vi "Current_Training_UI_3.10.22.vi"() -> ()   [LabVIEW 2019]
panel:
  out "Console out 2":string
  out "Console out":string
  out "intro":picture
  out "view":picture
  out "training 2":picture
  out "sent string":string
  out "training":u16[](array[numeric])
  out "Motor Value":i32
  in  "Quit":bool
  out "Training String":string
  out "Tab Control":enum32{"Welcome", "View", "Train"}(tab)
  in  "Ready":bool
  out "Motor Position View":u8(knob) scale=0.0..4.0
  in  "TRAIN":bool
  out "Sensor Intensity % View":dbl(slide) scale=0.0..100.0
  out "?":u32(colorbox)
  in  "Done":bool
  in  "Motor Position":u8(knob) scale=0.0..4.0
  out "Light Intensity %":dbl(slide) scale=0.0..100.0
  in  "Training Data":bool
  in  "Upload":bool
  out "Light Intensity 2":u32(colorbox)
  out "table":picture
  in  "Done 2":bool
  out "concatenated string":string
  out "read buffer":string
  out "Motor":string
  out "Sensor":string
  out "Type":string
  out "Name":string
  out "read terminal buffer - view":string
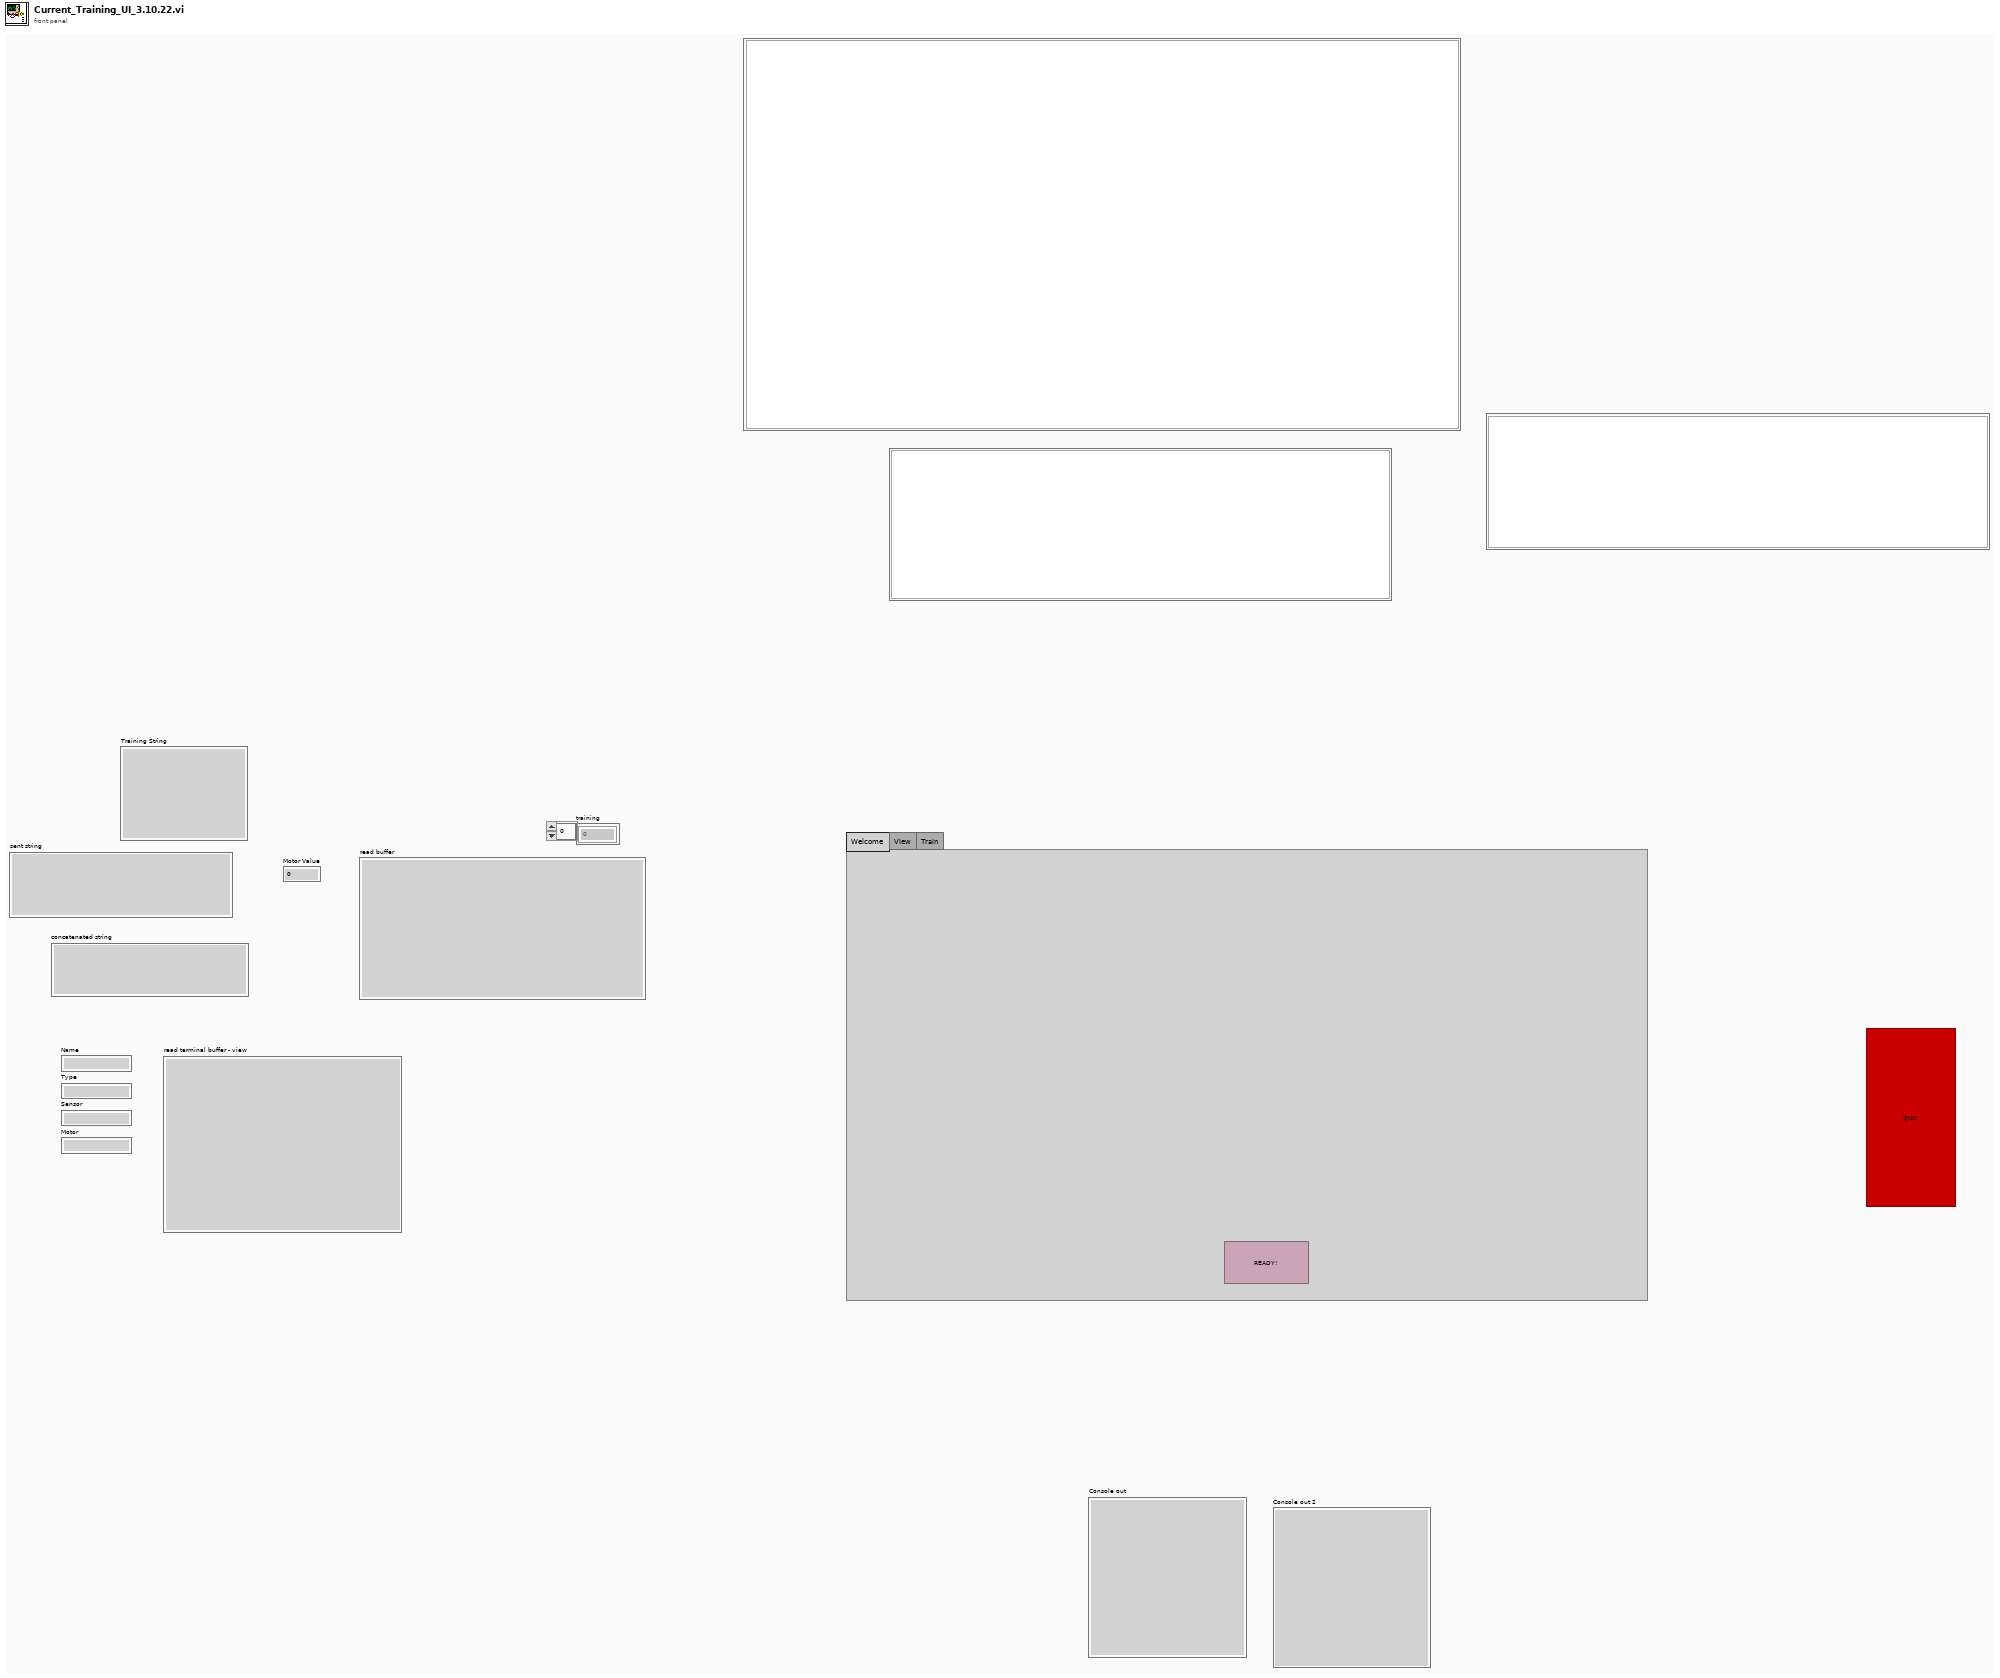
[diagram p1: front panel]
types:
  T1 = typedef "PythonCtrl.ctl" = cluster{"session":refnum<k35>, "PyPath":path, "Processor":enum16{"SPIKE", "Pi", "Pi_ssh"}}
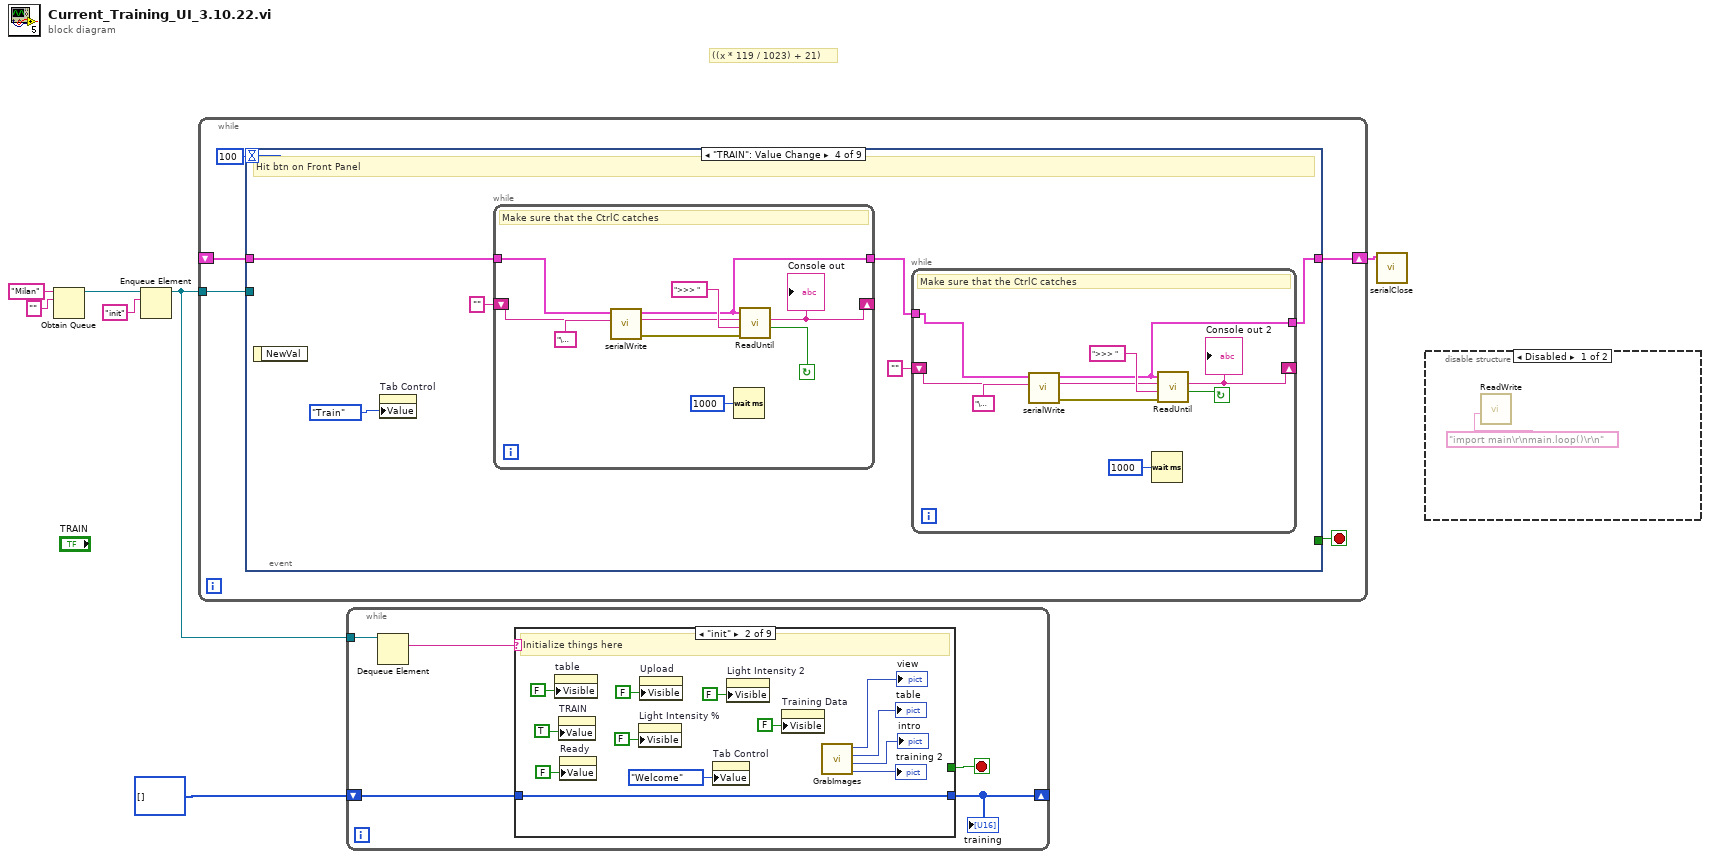
[diagram p0: block diagram]
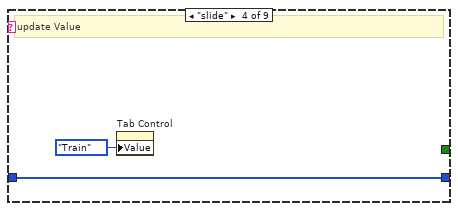
[diagram p5: hidden frame]
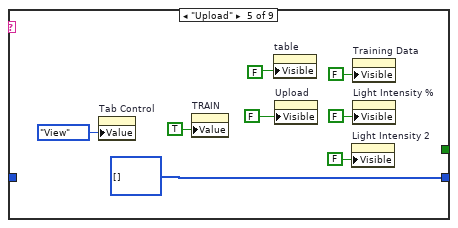
[diagram p6: hidden frame]
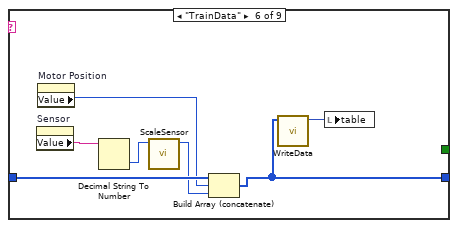
[diagram p7: hidden frame]
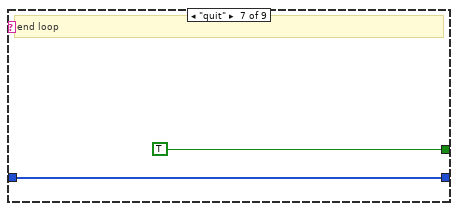
[diagram p8: hidden frame]
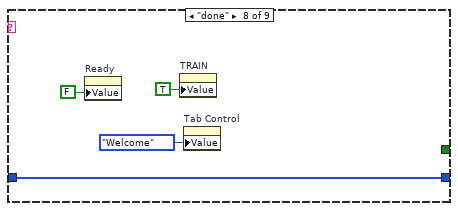
[diagram p9: hidden frame]
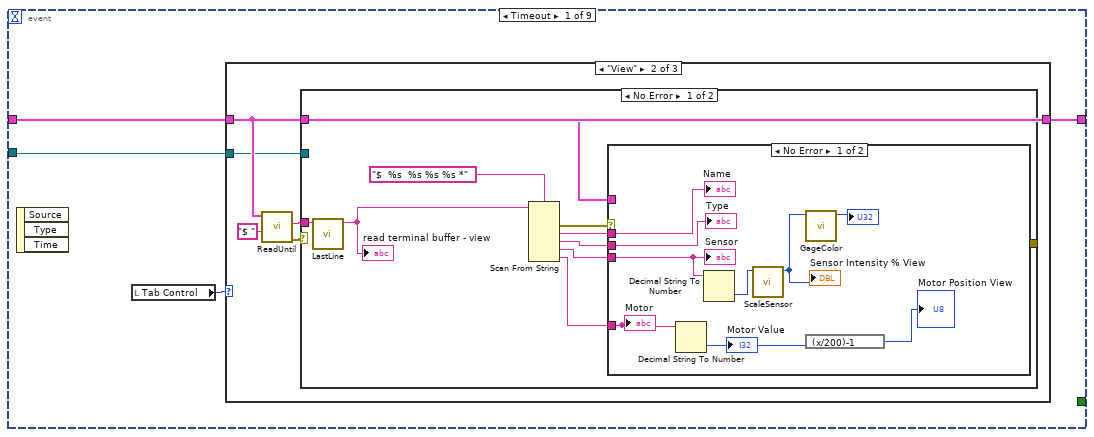
[diagram p11: hidden frame]
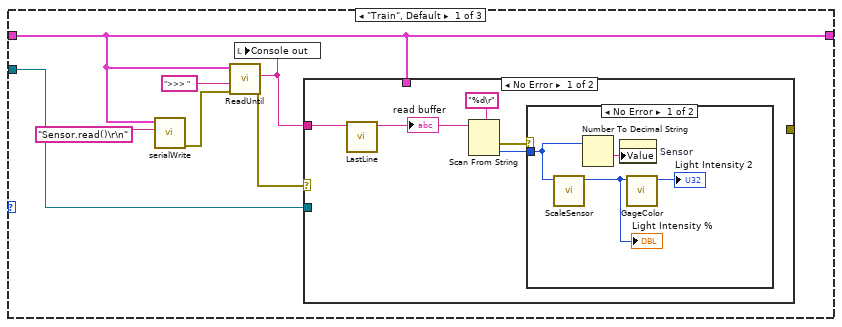
[diagram p12: hidden frame]
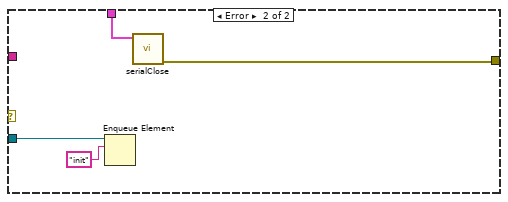
[diagram p14: hidden frame]
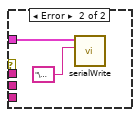
[diagram p15: hidden frame]
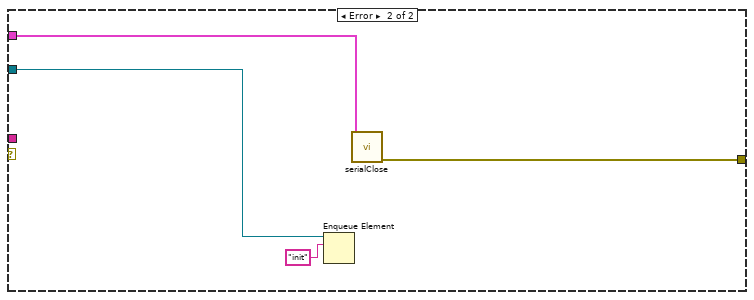
[diagram p16: hidden frame]
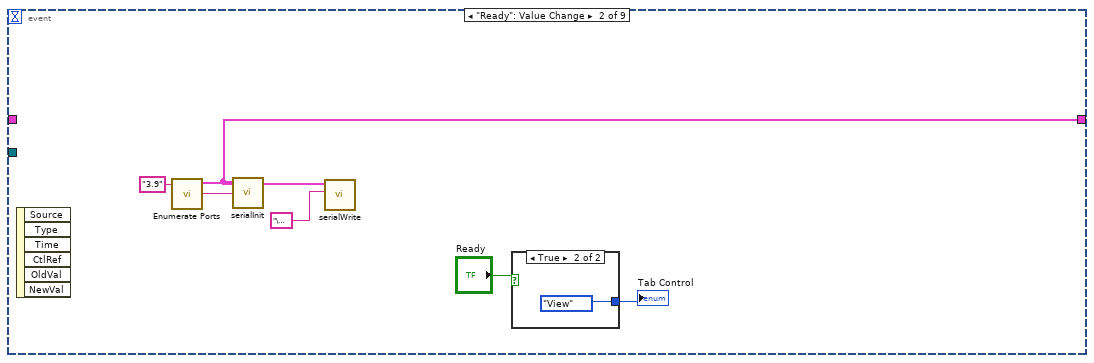
[diagram p18: hidden frame]
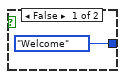
[diagram p19: hidden frame]
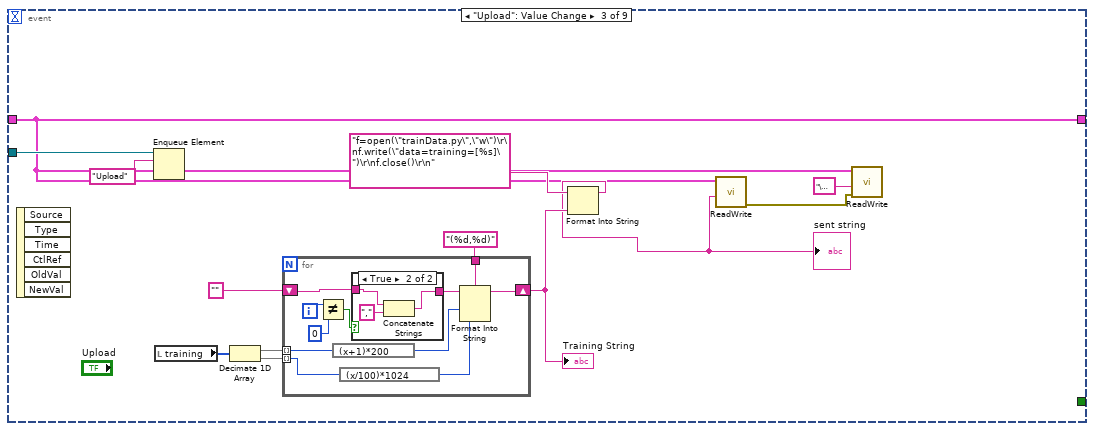
[diagram p20: hidden frame]
diagram:
  # "((x * 119 / 1023) + 21)"
  n1 = Obtain Queue(name (unnamed)="Milan", element data type="") -> (queue out=w7:refnum<queue>)  [unwired: 3 in, 2 out]
  n2 = Enqueue Element(queue=w7, element="init") -> (queue out=w3:refnum<queue>)  [unwired: 2 in, 2 out]
  n3 = while {
    tunnel: w3 -> [w12]
    shift-right: [w9] -> w2
    shift-left: _ -> [w10]
    stop <- w11 stop-if-true
    n4 = event shown="[3] \"TRAIN\": Value Change" {
      selector: _ -> [_ _ _ _ _ _ _ _ _]
      dyn-events: _ -> [_ _ _ _ _ _ _ _ _]
      timeout: 100 -> [_ _ _ _ _ _ _ _ _]
      tunnel: w12 -> [w13 _ w87 _ w128 w138 w142 w146 w150]
      tunnel: [_ _ _ _ _ _ w141 TRUE ("Discard?") _] -> w11
      tunnel: w10 -> [w15 _ w75 w107 w127 w137 w140 w144 w148]
      tunnel: [w16 w67 w75 w103 w127 w137 w140 w144 w148] -> w9
      tunnel: [_ _ w75 _ _ _ _ _ _] -> _
      event Timeout {
        n5 = event-data() -> ()  [unwired: 1 in, 3 out]
        n6 = local read "Tab Control"() -> (w14:enum32{"Welcome", "View", "Train"})
        n7 = case shown="\"View\"" w14 {
          tunnel: w15 -> [w18 w41 w66]
          tunnel: [w18 w41 w66] -> w16
          tunnel: w13 -> [w17 w37 _]
          frame "Train", Default {
            n8 = call "serialWrite.vi"("text"="Sensor.read()\r\n" ("write buffer"), "Python"=w18) -> ("error out"=w21:errorcluster)  [unwired: 8 in, 1 out]
            n9 = call "ReadUntil.vi"("error in (no error)"=w21, "EOL"=">>> ", "Python"=w18) -> ("error out"=w19:errorcluster, "Console out"=w20:string)  [unwired: 6 in, 1 out]
            n10 = local write "Console out"(w20) -> ()
            n11 = case shown="No Error" w19 {
              tunnel: w20 -> [w24 _]
              tunnel: w18 -> [_ w35]
              tunnel: w17 -> [_ w34]
              tunnel: [_ w33] -> _
              frame No Error {
                n12 = call "LastLine.vi"("Reply"=w24) -> ("String"=w25:string)  [unwired: 10 in]
                "read buffer" <- w25
                n13 = Scan From String(format string="%d\r", input string=w25) -> (error out=w28:errorcluster, output 1=w27:i32)  [unwired: 3 in, 2 out]
                n14 = case shown="No Error" w28 {
                  tunnel: w27 -> [w30 _]
                  frame No Error {
                    n15 = call "ScaleSensor.vi"("value"=w30) -> ("scaled value"=w29:u16)  [unwired: 10 in]
                    "Light Intensity %" <- w29
                    n16 = Number To Decimal String(number=w30) -> (decimal integer string=w32:string)  [unwired: 1 in]
                    n17 = property on="Sensor" class="Str"("Value"=w32) -> ()  [unwired: 2 in, 2 out]
                    n18 = call "GageColor.vi"("value"=w29) -> ("Color Box"=→"Light Intensity 2":u32)  [unwired: 10 in]
                  }
                  frame Error {
                  }
                }
              }
              frame Error {
                n19 = Enqueue Element(queue=w34, element="init") -> ()  [unwired: 2 in, 3 out]
                n20 = call "serialClose.vi"("Python in"=w35) -> ("error out"=w33:errorcluster)  [unwired: 10 in]
              }
            }
          }
          frame "View" {
            n21 = call "ReadUntil.vi"("EOL"="$ ", "Python"=w41) -> ("error out"=w39:errorcluster, "Console out"=w40:string)  [unwired: 7 in, 1 out]
            n22 = case shown="No Error" w39 {
              tunnel: w40 -> [w44 _]
              tunnel: w41 -> [w42 w64]
              tunnel: w37 -> [_ w63]
              tunnel: [_ w62] -> _
              frame No Error {
                n23 = call "LastLine.vi"("Reply"=w44) -> ("String"=w43:string)  [unwired: 10 in]
                "read terminal buffer - view" <- w43
                n24 = Scan From String(format string="$  %s  %s %s %s *", input string=w43) -> (error out=w50:errorcluster, output 1=w46:string, output 2=w47:string, output 3=w48:string, output 4=w49:string)  [unwired: 6 in, 2 out]
                n25 = case shown="No Error" w50 {
                  tunnel: w46 -> [w59 _]
                  tunnel: w47 -> [w58 _]
                  tunnel: w48 -> [w57 _]
                  tunnel: w49 -> [w54 _]
                  tunnel: w42 -> [_ w61]
                  frame No Error {
                    n26 = Decimal String To Number(string=w54) -> (number=w52:i32)  [unwired: 2 in, 1 out]
                    "Motor Value" <- w52
                    n27 = Decimal String To Number(string=w57) -> (number=w56:i32)  [unwired: 2 in, 1 out]
                    n28 = call "ScaleSensor.vi"("value"=w56) -> ("scaled value"=w53:u16)  [unwired: 10 in]
                    "Sensor Intensity % View" <- w53
                    n29 = call "GageColor.vi"("value"=w53) -> ("Color Box"=→"?":u32)  [unwired: 10 in]
                    n30 = expression code="(x/200)-1"(w52) -> (→"Motor Position View":i32)
                    "Name" <- w59
                    "Type" <- w58
                    "Sensor" <- w57
                    "Motor" <- w54
                  }
                  frame Error {
                    n31 = call "serialWrite.vi"("text"="\u0003", "Python"=w61) -> ()  [unwired: 8 in, 2 out]
                  }
                }
              }
              frame Error {
                n32 = Enqueue Element(queue=w63, element="init") -> ()  [unwired: 2 in, 3 out]
                n33 = call "serialClose.vi"("Python in"=w64) -> ("error out"=w62:errorcluster)  [unwired: 10 in]
              }
            }
          }
          frame "Welcome" {
          }
        }
      }
      event "Ready": Value Change {
        n34 = event-data() -> ()  [unwired: 1 in, 6 out]
        n35 = call "Enumerate Ports.vi"("Python version"="3.9") -> ("guess"=w70:string, "Python"=w67:T1)  [unwired: 6 in, 3 out]
        n36 = call "serialInit.vi"("Port"=w70, "Python"=w67) -> ()  [unwired: 8 in, 2 out]
        n37 = call "serialWrite.vi"("text"="\u0004" ("write buffer"), "Python"=w67) -> ()  [unwired: 8 in, 2 out]
        n38 = case shown="True" "Ready" {
          tunnel: [enum32{"Welcome", "View", "Train"}."Welcome" ("Tab Control") enum32{"Welcome", "View", "Train"}."View" ("Tab Control")] -> w71
          frame False {
          }
          frame True {
          }
        }
        "Tab Control" <- w71
      }
      event "Upload": Value Change {
        n39 = event-data() -> ()  [unwired: 1 in, 6 out]
        n40 = Enqueue Element(queue=w87, element="Upload") -> ()  [unwired: 2 in, 3 out]
        n41 = local read "training"() -> (w85:u16[])
        n42 = Decimate 1D Array(w85) -> (w83:u16[], w82:u16[])
        n43 = for {
          tunnel: "(%d,%d)" ("format string") -> [w98]
          tunnel: w83 -> [w91] mode=indexing
          tunnel: w82 -> [w89] mode=indexing
          shift-right: [w97] -> w80
          shift-left: "" -> [w96]
          i -> [w93]
          n44 = Not Equal?(x=w93, y=0) -> (x != y?=w94:bool)
          n45 = expression code="(x+1)*200"(w91) -> (w90:u16)
          n46 = expression code="(x/100)*1024"(w89) -> (w88:u16)
          n47 = case shown="True" w94 {
            tunnel: w96 -> [w99 w101]
            tunnel: [w99 w100] -> w95
            frame False {
            }
            frame True {
              n48 = Concatenate Strings(w101, "," ("string")) -> (w100:string)
            }
          }
          n49 = Format Into String(format string=w98, initial string=w95, w90, w88) -> (resulting string=w97:string)  [unwired: 1 in, 1 out]
        }
        "Training String" <- w80
        n50 = Format Into String(format string="f=open(\"trainData.py\",\"w\")\r\nf.write(\"data=training=[%s]\")\r\nf.close()\r\n" ("string"), w80) -> (resulting string=w78:string)  [unwired: 2 in, 1 out]
        "sent string" <- w78
        n51 = call "ReadWrite.vi"("Code"=w78, "Python"=w75) -> ("error out"=w76:errorcluster)  [unwired: 8 in, 1 out]
        n52 = call "ReadWrite.vi"("error in (no error)"=w76, "Code"="\u0004" ("text"), "Python"=w75) -> ()  [unwired: 7 in, 2 out]
      }
      event "TRAIN": Value Change {
        # "Hit btn on Front Panel"
        n53 = event-data() -> ()  [unwired: 1 in, 1 out]
        n54 = property on="Tab Control" class="TabCtl (strict)"("Value"=enum32{"Welcome", "View", "Train"}."Train" ("Tab Control")) -> ()  [unwired: 2 in, 2 out]
        n55 = while {
          tunnel: w107 -> [w119]
          tunnel: [w119] -> w104
          shift-right: [w118] -> _
          shift-left: "" ("Console out") -> [w117]
          stop <- w121 continue-if-true
          # "Make sure that the CtrlC catches"
          n56 = call "serialWrite.vi"("text"="\u0003" ("write buffer"), "Python"=w119) -> ("error out"=w122:errorcluster)  [unwired: 8 in, 1 out]
          n57 = Wait (ms)(milliseconds to wait=u32 1000) -> ()  [unwired: 1 out]
          n58 = call "ReadUntil.vi"("error in (no error)"=w122, "EOL"=">>> ", "Console in"=w117, "Python"=w119) -> ("timed out?"=w121:bool, "Console out"=w118:string)  [unwired: 5 in, 1 out]
          "Console out" <- w118
        }
        n59 = while {
          tunnel: [w109] -> w103
          shift-right: [w111] -> _
          shift-left: "" ("Console out") -> [w110]
          tunnel: w104 -> [w109]
          stop <- w113 continue-if-true
          # "Make sure that the CtrlC catches"
          n60 = call "serialWrite.vi"("text"="\u0003" ("write buffer"), "Python"=w109) -> ("error out"=w114:errorcluster)  [unwired: 8 in, 1 out]
          n61 = Wait (ms)(milliseconds to wait=u32 1000) -> ()  [unwired: 1 out]
          n62 = call "ReadUntil.vi"("error in (no error)"=w114, "EOL"=">>> ", "Console in"=w110, "Python"=w109) -> ("timed out?"=w113:bool, "Console out"=w111:string)  [unwired: 5 in, 1 out]
          "Console out 2" <- w111
        }
      }
      event "Training Data": Value Change {
        n63 = event-data() -> ()  [unwired: 1 in, 6 out]
        n64 = Enqueue Element(queue=w128, element="TrainData") -> ()  [unwired: 2 in, 3 out]
        n65 = property on="table" class="Pict"("Visible"=TRUE) -> ()  [unwired: 2 in, 2 out]
        n66 = property on="Upload" class="Bool (strict)"("Visible"=TRUE) -> ()  [unwired: 2 in, 2 out]
      }
      event "Motor Position": Value Change {
        # "Slide slid on Front Panel"
        n67 = event-data() -> ()  [unwired: 1 in, 6 out]
        n68 = Enqueue Element(queue=w138, element="slide") -> ()  [unwired: 2 in, 3 out]
        n69 = property on="Training Data" class="Bool"("Visible"=TRUE) -> ()  [unwired: 2 in, 2 out]
        n70 = expression code="(x+1)*30"("Motor Position") -> (w133:u8)
        n71 = Format Into String(format string="pwm2.duty(%d)\r\n", w133) -> (resulting string=w135:string)  [unwired: 2 in, 1 out]
        "concatenated string" <- w135
        n72 = property on="Light Intensity %" class="Slide (strict)"("Visible"=TRUE) -> ()  [unwired: 2 in, 2 out]
        n73 = call "serialWrite.vi"("text"=w135, "Python"=w137) -> ()  [unwired: 8 in, 2 out]
        n74 = property on="Light Intensity 2" class="ColBox"("Visible"=TRUE) -> ()  [unwired: 2 in, 2 out]
      }
      event Panel Close? {
        w141 = TRUE ("Discard?")
        # "Closed the Window"
        n75 = event-data() -> ()  [unwired: 1 in, 2 out]
        n76 = Enqueue Element(queue=w142, element="done") -> ()  [unwired: 2 in, 3 out]
        n77 = event-data("Discard?"=w141) -> ()  [unwired: 1 in, 1 out]
      }
      event "Quit": Value Change {
        # "hit Done btn"
        n78 = event-data() -> ()  [unwired: 1 in, 2 out]
        n79 = Enqueue Element(queue=w146, element="quit") -> ()  [unwired: 2 in, 3 out]
      }
      event "Done", "Done 2": Value Change {
        n80 = event-data() -> ()  [unwired: 1 in, 6 out]
        n81 = Enqueue Element(queue=w150, element="done") -> ()  [unwired: 2 in, 3 out]
        n82 = call "ReadWrite.vi"("Code"="\u0004" ("text"), "Python"=w148) -> ()  [unwired: 8 in, 2 out]
      }
    }
  }
  n83 = while {
    tunnel: w3 -> [w156]
    shift-right: [w152] -> _
    shift-left: u16[] [] ("initialized array") -> [w153]
    stop <- w154 stop-if-true
    n84 = Dequeue Element(queue=w156) -> (element=w155:string)  [unwired: 2 in, 3 out]
    n85 = case shown="\"init\"" w155 {
      tunnel: [_ _ _ _ _ _ TRUE ("Discard?") _ _] -> w154
      tunnel: w153 -> [w157 w170 w171 w173 _ w188 w189 w193 w195]
      tunnel: [w157 w170 w171 w173 u16[] [] ("initialized array") w184 w189 w193 w195] -> w152
      frame Default {
      }
      frame "init" {
        # "Initialize things here"
        n86 = property on="table" class="Pict"("Visible"=FALSE) -> ()  [unwired: 2 in, 2 out]
        n87 = property on="TRAIN" class="Bool (strict)"("Value"=TRUE ("Train")) -> ()  [unwired: 2 in, 2 out]
        n88 = property on="Ready" class="Bool (strict)"("Value"=FALSE ("Ready")) -> ()  [unwired: 2 in, 2 out]
        n89 = property on="Light Intensity %" class="Slide (strict)"("Visible"=FALSE) -> ()  [unwired: 2 in, 2 out]
        n90 = property on="Upload" class="Bool (strict)"("Visible"=FALSE) -> ()  [unwired: 2 in, 2 out]
        n91 = property on="Tab Control" class="TabCtl (strict)"("Value"=enum32{"Welcome", "View", "Train"}."Welcome" ("Tab Control")) -> ()  [unwired: 2 in, 2 out]
        n92 = property on="Light Intensity 2" class="ColBox"("Visible"=FALSE) -> ()  [unwired: 2 in, 2 out]
        n93 = property on="Training Data" class="Bool"("Visible"=FALSE) -> ()  [unwired: 2 in, 2 out]
        n94 = call "GrabImages.vi"() -> ("Training Instructions"=→"training 2":picture, "Intro"=→"intro":picture, "Table"=→"table":picture, "View Instructions"=→"view":picture)  [unwired: 8 in]
      }
      frame "Train" {
        # "reset LED"
      }
      frame "slide" {
        # "update Value"
        n95 = property on="Tab Control" class="TabCtl (strict)"("Value"=enum32{"Welcome", "View", "Train"}."Train" ("Tab Control")) -> ()  [unwired: 2 in, 2 out]
      }
      frame "Upload" {
        n96 = property on="Tab Control" class="TabCtl (strict)"("Value"=enum32{"Welcome", "View", "Train"}."View" ("Tab Control")) -> ()  [unwired: 2 in, 2 out]
        n97 = property on="TRAIN" class="Bool (strict)"("Value"=TRUE ("TRAIN")) -> ()  [unwired: 2 in, 2 out]
        n98 = property on="table" class="Pict"("Visible"=FALSE) -> ()  [unwired: 2 in, 2 out]
        n99 = property on="Upload" class="Bool (strict)"("Visible"=FALSE) -> ()  [unwired: 2 in, 2 out]
        n100 = property on="Light Intensity 2" class="ColBox"("Visible"=FALSE) -> ()  [unwired: 2 in, 2 out]
        n101 = property on="Training Data" class="Bool"("Visible"=FALSE) -> ()  [unwired: 2 in, 2 out]
        n102 = property on="Light Intensity %" class="Slide (strict)"("Visible"=FALSE) -> ()  [unwired: 2 in, 2 out]
      }
      frame "TrainData" {
        n103 = property on="Sensor" class="Str"() -> ("Value"=w187:string)  [unwired: 2 in, 2 out]
        n104 = property on="Motor Position" class="Knob (strict)"() -> ("Value"=w182:u8)  [unwired: 2 in, 2 out]
        n105 = Decimal String To Number(string=w187) -> (number=w186:i32)  [unwired: 2 in, 1 out]
        n106 = call "ScaleSensor.vi"("value"=w186) -> ("scaled value"=w185:u16)  [unwired: 10 in]
        n107 = Build Array (concatenate)(w188, w182, w185) -> (w184:u16[])
        n108 = call "WriteData.vi"("Array"=w184) -> ("Table"=w183:picture)  [unwired: 10 in]
        n109 = local write "table"(w183) -> ()
      }
      frame "quit" {
        # "end loop"
      }
      frame "done" {
        n110 = property on="Ready" class="Bool (strict)"("Value"=FALSE ("Ready")) -> ()  [unwired: 2 in, 2 out]
        n111 = property on="TRAIN" class="Bool (strict)"("Value"=TRUE ("TRAIN")) -> ()  [unwired: 2 in, 2 out]
        n112 = property on="Tab Control" class="TabCtl (strict)"("Value"=enum32{"Welcome", "View", "Train"}."Welcome" ("Tab Control")) -> ()  [unwired: 2 in, 2 out]
      }
      frame "" {
      }
    }
    "training" <- w152
  }
  n113 = call "serialClose.vi"("Python in"=w2) -> ()  [unwired: 10 in, 1 out]
  n114 = disable-structure shown="Disabled" {
    frame Disabled {
      n115 = call "ReadWrite.vi"("Code"="import main\r\nmain.loop()\r\n" ("text")) -> ()  [unwired: 9 in, 2 out]
    }
    frame Enabled {
    }
  }
